vi "Check.vi"(8 "error in (no error)":errorcluster, 11 "Watchdog in":refnum<class "Watchdog.lvclass">) -> (0 "error out":errorcluster, 1 "Watchdog Name":string, 2 "Expired":bool, 3 "Watchdog out":refnum<class "Watchdog.lvclass">, 5 "Execution Timeout":u32)   [LabVIEW 2017, in "Watchdog.lvclass"]
doc: "Check if the watchdog has expired."
uses:
  <vilib>/NI/Software Watchdog/Watchdog/Watchdog.lvclass
  <vilib>/NI/Software Watchdog/Watchdog/Watchdog.lvclass/Watchdog.ctl
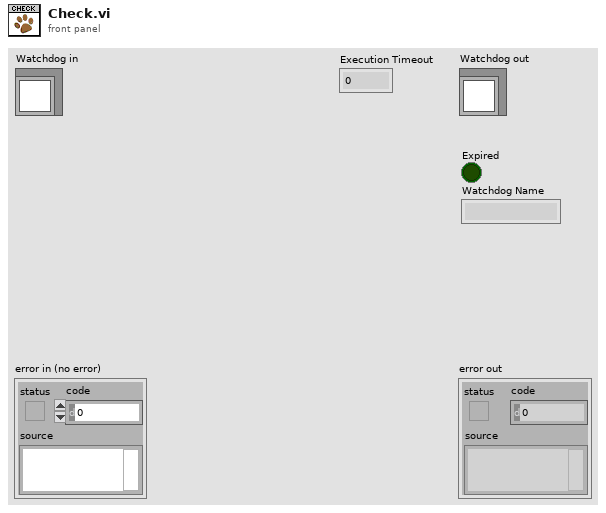
[diagram p1: front panel]
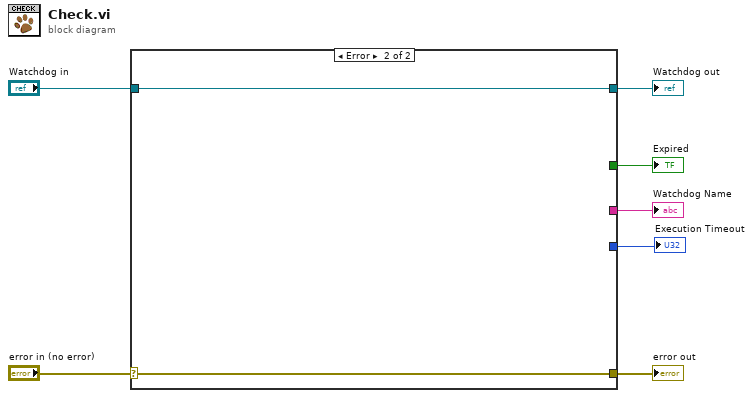
[diagram p0: block diagram]
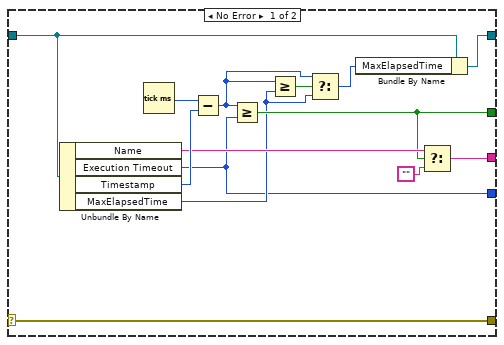
[diagram p2: hidden frame]
diagram:
  n1 = case shown="Error" "error in (no error)" {
    selector: "error in (no error)" -> [w21 w23]
    tunnel: [w21 w23] -> w6
    tunnel: [w13 w22] -> w4
    tunnel: "Watchdog in" -> [w14 w22]
    tunnel: [w16 _] -> w2
    tunnel: [w15 _] -> w3
    tunnel: [w8 _] -> w1
    frame No Error {
      n2 = Unbundle By Name(w14) -> ("Name"=w18:string, "Execution Timeout"=w8:u32, "Timestamp"=w19:u32, "MaxElapsedTime"=w10:u32)
      n3 = Tick Count (ms)() -> (millisecond timer value=w20:u32)
      n4 = Subtract(x=w20, y=w19) -> (x-y=w11:u32)
      n5 = Greater Or Equal?(x=w11, y=w8) -> (x >= y?=w15:bool)
      n6 = Greater Or Equal?(x=w11, y=w10) -> (x >= y?=w12:bool)
      n7 = Select(t=w11, s=w12, f=w10) -> (s? t:f=w9:u32)
      n8 = Bundle By Name(cluster=w14, "MaxElapsedTime"=w9) -> (w13:refnum<class "Watchdog.lvclass">)
      n9 = Select(t=w18, s=w15, f="") -> (s? t:f=w16:string)
    }
    frame Error {
    }
  }
  "error out" <- w6
  "Watchdog out" <- w4
  "Expired" <- w3
  "Watchdog Name" <- w2
  "Execution Timeout" <- w1
